vi "CreatePanes.vi"(8 "error in":errorcluster, 11 "PythonConverter_GUI in":refnum<class "PythonConverter_GUI.lvclass">) -> (0 "error out":errorcluster, 3 "PythonConverter_GUI out":refnum<class "PythonConverter_GUI.lvclass">, 6 "panes":string[](array[string]))   [LabVIEW 2014, in "Raspberry Pi Compatible Compiler for LabVIEW.lvlib" / "PythonConverter_GUI.lvclass"]
uses:
  PythonConverter_GUI.lvclass
  PythonConverter_GUI.lvclass/PythonConverter_GUI.ctl
  Parsing/ClassTypeTD.ctl
  VI Interpreter/Classes/Pane/Pane.lvclass
  VI Interpreter/Classes/VI Interpreter/VI Interpreter.lvclass
  Parsing/Python Functions.lvlib
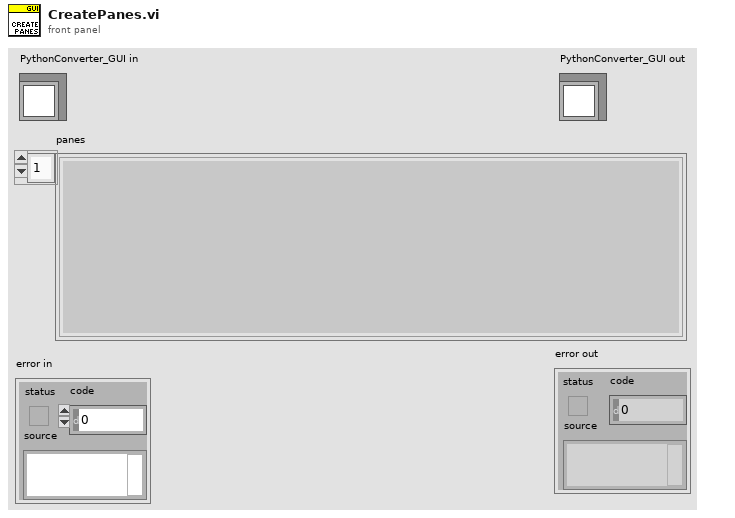
[diagram p1: front panel]
types:
  T1 = typedef "Raspberry Pi Compatible Compiler for LabVIEW.lvlib/Python Functions.lvlib/ClassTypeTD.ctl" = enum16{"class", "function"}
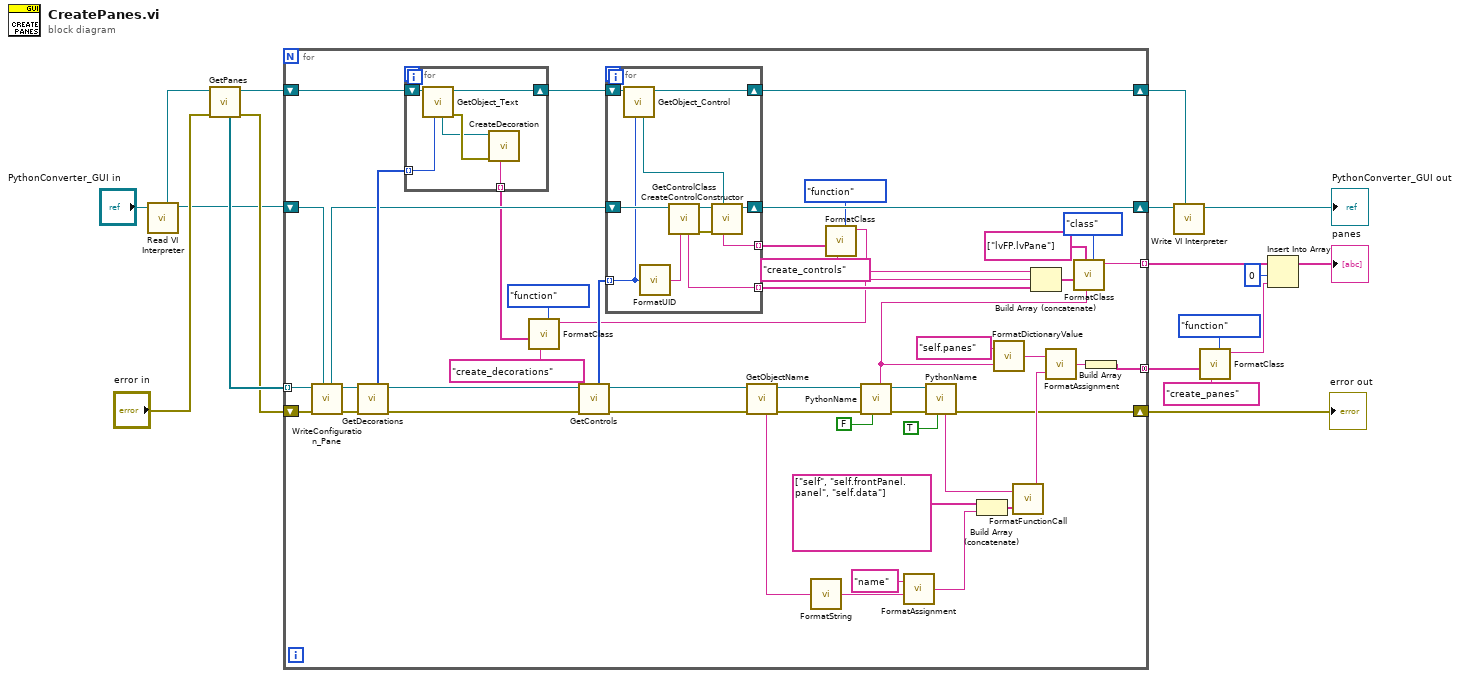
[diagram p0: block diagram]
diagram:
  n1 = call "Read VI Interpreter.vi"("PythonConverter_GUI in"="PythonConverter_GUI in") -> ("PythonConverter_GUI out"=w9:refnum<class "PythonConverter_GUI.lvclass">, "VI Interpreter"=w10:refnum<class "VI Interpreter.lvclass">)  [unwired: 7 in]
  n2 = call "GetPanes.vi"("error in"="error in", "VI Interpreter in"=w10) -> ("error out"=w16:errorcluster, "VI Interpreter out"=w6:refnum<class "VI Interpreter.lvclass">, "Panes"=w17:refnum<class "Pane.lvclass">[])  [unwired: 5 in]
  n3 = for {
    tunnel: w17 -> [w59] mode=indexing
    shift-right: [w38] -> w13
    shift-left: w16 -> [w58]
    tunnel: [w60] -> w12 mode=concatenating
    shift-right: [w54] -> w8
    shift-left: w9 -> [w57]
    tunnel: [w51] -> w4 mode=indexing
    shift-right: [w48] -> w5
    shift-left: w6 -> [w27]
    n4 = call "WriteConfiguration_Pane.vi"("PythonConverter_GUI in"=w57, "error in"=w58, "Pane in"=w59) -> ("error out"=w29:errorcluster, "Pane out"=w31:refnum<class "Pane.lvclass">, "PythonConverter_GUI out"=w24:refnum<class "PythonConverter_GUI.lvclass">)  [unwired: 6 in]
    n5 = call "GetDecorations.vi"("error in"=w29, "Pane in"=w31) -> ("error out"=w28:errorcluster, "Pane out"=w30:refnum<class "Pane.lvclass">, "decorations"=w25:i32[])  [unwired: 5 in]
    n6 = for {
      tunnel: w25 -> [w72] mode=indexing
      shift-right: [w68] -> w26
      shift-left: w27 -> [w73]
      tunnel: [w69] -> w22 mode=indexing
      n7 = call "GetObject_Text.vi"("UID"=w72, "VI Interpreter in"=w73) -> ("error out"=w71:errorcluster, "VI Interpreter out"=w68:refnum<class "VI Interpreter.lvclass">, "Text"=w70:refnum<class "Text.lvclass">)  [unwired: 4 in, 1 out]
      n8 = call "CreateDecoration.vi"("error in"=w71, "Decoration in"=w70) -> ("decoration"=w69:string)  [unwired: 6 in, 3 out]
    }
    n9 = call "FormatClass.vi"("type"=ClassTypeTD."function", "name"="create_decorations", "body"=w22) -> ("python"=w19:string)  [unwired: 8 in]
    n10 = call "GetControls.vi"("error in"=w28, "Pane in"=w30) -> ("error out"=w34:errorcluster, "Pane out"=w49:refnum<class "Pane.lvclass">, "Controls"=w50:i32[])  [unwired: 5 in]
    n11 = for {
      shift-right: [w77] -> w54
      shift-left: w24 -> [w82]
      tunnel: [w84] -> w44 mode=indexing
      tunnel: w50 -> [w80] mode=indexing
      shift-right: [w75] -> w48
      shift-left: w26 -> [w81]
      tunnel: [w79] -> w46 mode=indexing
      n12 = call "GetObject_Control.vi"("UID"=w80, "VI Interpreter in"=w81) -> ("VI Interpreter out"=w75:refnum<class "VI Interpreter.lvclass">, "control"=w76:refnum<class "Control.lvclass">)  [unwired: 4 in, 2 out]
      n13 = call "FormatUID.vi"("UID"=w80) -> ("Name"=w83:string)
      n14 = call "GetControlClass.vi"("name"=w83, "PythonConverter_GUI in"=w82) -> ("error out"=w74:errorcluster, "PythonConverter_GUI out"=w78:refnum<class "PythonConverter_GUI.lvclass">, "class"=w84:string)  [unwired: 5 in]
      n15 = call "CreateControlConstructor.vi"("Control in"=w76, "error in"=w74, "PythonConverter_GUI in"=w78) -> ("PythonConverter_GUI out"=w77:refnum<class "PythonConverter_GUI.lvclass">, "control"=w79:string)  [unwired: 4 in, 3 out]
    }
    n16 = call-dynamic "GetObjectName.vi"("error in"=w34, "GObject in"=w49) -> ("error out"=w35:errorcluster, "GObject out"=w36:refnum<class "Pane.lvclass">, "Name"=w56:string)  [unwired: 5 in]
    n17 = call "FormatString.vi"("value"=w56) -> ("python object"=w55:string)
    n18 = call "FormatClass.vi"("type"=ClassTypeTD."function", "name"="create_controls", "body"=w46) -> ("python"=w20:string)  [unwired: 8 in]
    n19 = call-dynamic "PythonName.vi"("add self"=FALSE, "error in"=w35, "Pane in"=w36) -> ("error out"=w37:errorcluster, "Pane out"=w39:refnum<class "Pane.lvclass">, "name"=w41:string)  [unwired: 5 in, 1 out]
    n20 = call "FormatAssignment.vi"("value"=w55, "name"="name") -> ("python assignment"=w62:string)
    n21 = call-dynamic "PythonName.vi"("add self"=TRUE, "error in"=w37, "Pane in"=w39) -> ("error out"=w38:errorcluster, "name"=w42:string)  [unwired: 5 in, 2 out]
    n22 = Build Array (concatenate)(string[] ["self", "self.frontPanel.panel", "self.data"] ("parameters"), w62) -> (w61:string[])
    n23 = call "FormatDictionaryValue.vi"("key"=w41, "dictionary"="self.panes") -> ("python object"=w40:string)
    n24 = call "FormatFunctionCall.vi"("parameters"=w61, "function"=w42) -> ("python object"=w65:string)
    n25 = Build Array (concatenate)(w20, w19, w44) -> (w43:string[])
    n26 = call "FormatAssignment.vi"("value"=w65, "name"=w40) -> ("python assignment"=w66:string)
    n27 = call "FormatClass.vi"("type"=ClassTypeTD."class", "name"=w41, "parameters/ancestors"=string[] ["lvFP.lvPane"], "body"=w43) -> ("python"=w51:string)  [unwired: 7 in]
    n28 = Build Array(w66) -> (w60:string[])
  }
  "error out" <- w13
  n29 = call "Write VI Interpreter.vi"("VI Interpreter"=w5, "PythonConverter_GUI in"=w8) -> ("PythonConverter_GUI out"=→"PythonConverter_GUI out":refnum<class "PythonConverter_GUI.lvclass">)  [unwired: 7 in]
  n30 = call "FormatClass.vi"("type"=ClassTypeTD."function", "name"="create_panes", "body"=w12) -> ("python"=w2:string)  [unwired: 8 in]
  n31 = Insert Into Array(array=w4, index=0, new element=w2) -> (→"panes":string[])
